vi "oa_Get DSA 9232 Oversample Rate and Filter Delay.vi"(11 "Requested Sample Rate":dbl) -> (0 "Decimation Rate":u16, 1 "Input Delay":dbl, 2 "Internal Master Timebase":dbl=13107200.0, 3 "Actual Sample Rate":dbl)   [LabVIEW 2017, in "SoundVib_TachProcess.lvlib"]
uses:
  <vilib>/addons/Sound and Vibration/Order Analysis/Tach Process/SoundVib_TachProcess.lvlib
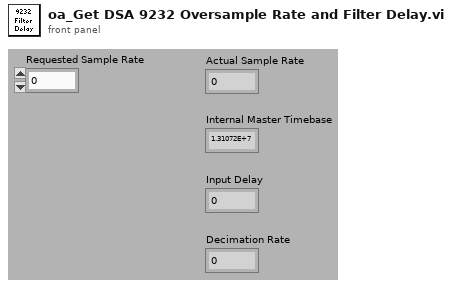
[diagram p1: front panel]
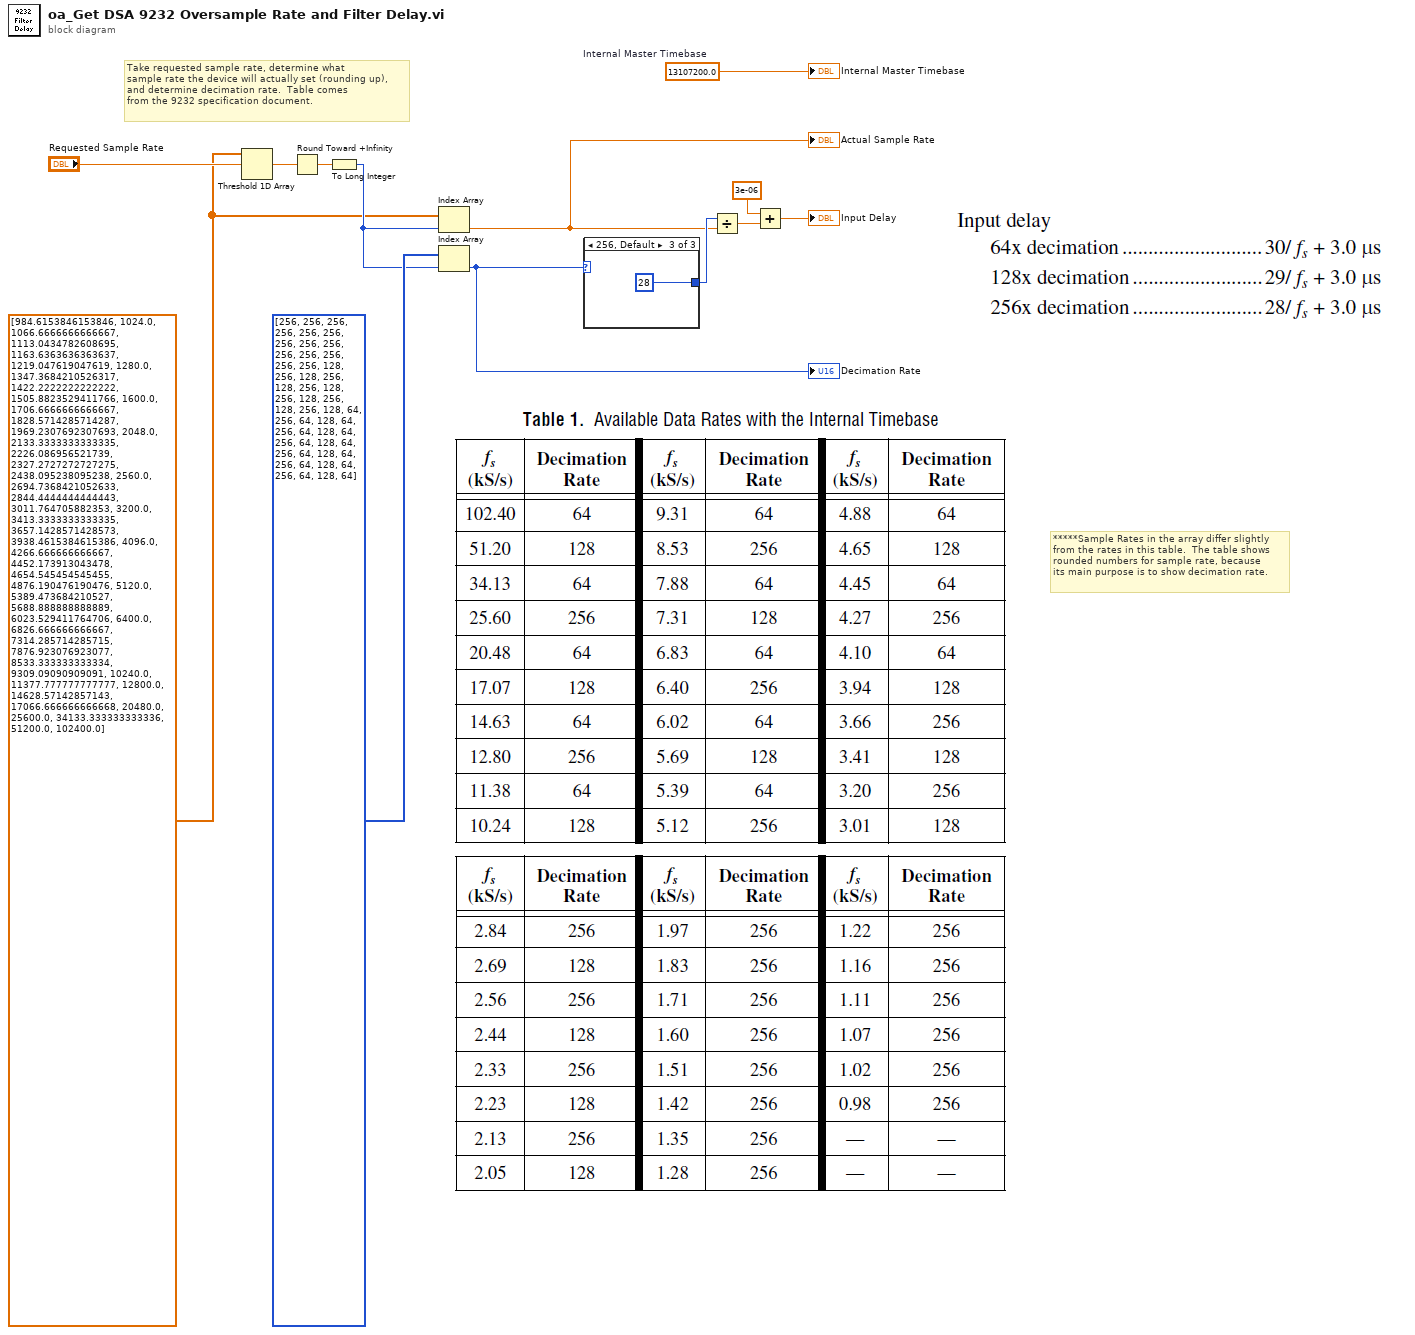
[diagram p0: block diagram]
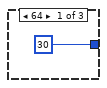
[diagram p2: hidden frame]
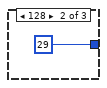
[diagram p3: hidden frame]
diagram:
  w1 = dbl[] [984.6153846153846, 1024.0, 1066.6666666666667, 1113.0434782608695, 1163.6363636363637, 1219.047619047619, 1280.0, 1347.3684210526317, 1422.2222222222222, 1505.8823529411766, 1600.0, 1706.6666666666667, 1828.5714285714287, 1969.2307692307693, 2048.0, 2133.3333333333335, 2226.086956521739, 2327.2727272727275, 2438.095238095238, 2560.0, 2694.7368421052633, 2844.4444444444443, 3011.764705882353, 3200.0, 3413.3333333333335, 3657.1428571428573, 3938.4615384615386, 4096.0, 4266.666666666667, 4452.173913043478, 4654.545454545455, 4876.190476190476, 5120.0, 5389.473684210527, 5688.888888888889, 6023.529411764706, 6400.0, 6826.666666666667, 7314.285714285715, 7876.923076923077, 8533.333333333334, 9309.09090909091, 10240.0, 11377.777777777777, 12800.0, 14628.57142857143, 17066.666666666668, 20480.0, 25600.0, 34133.333333333336, 51200.0, 102400.0] ("Possible Sample Rates")
  w2 = 13107200.0  # Internal Master Timebase
  # "*****Sample Rates in the array differ slightly\nfrom the rates in this table.  The table shows \nrounded numbers for sample rate, because\nits main purpose is to show decimation rate."
  # "Take requested sample rate, determine what\nsample rate the device will actually set (rounding up),\nand determine decimation rate.  Table comes\nfrom the 9232 specification document."
  n1 = Threshold 1D Array(2:"Requested Sample Rate", 3:w1) -> (0:w12:dbl)  [unwired: 1 in]
  n2 = Round Toward +Infinity(x=w12) -> (ceil(x): smallest int >= x=w10:dbl)
  n3 = To Long Integer(number=w10) -> (32bit integer=w9:i32)
  n4 = Index Array(array=w1, index=w9) -> (element=w6:dbl)
  "Actual Sample Rate" <- w6
  n5 = Index Array(array=u16[] [256, 256, 256, 256, 256, 256, 256, 256, 256, 256, 256, 256, 256, 256, 128, 256, 128, 256, 128, 256, 128, 256, 128, 256, 128, 256, 128, 64, 256, 64, 128, 64, 256, 64, 128, 64, 256, 64, 128, 64, 256, 64, 128, 64, 256, 64, 128, 64, 256, 64, 128, 64] ("reversed array"), index=w9) -> (element=w8:u16)
  "Decimation Rate" <- w8
  n6 = case shown="256, Default" w8 {
    tunnel: [30 29 28] -> w7
    frame 64 {
    }
    frame 128 {
    }
    frame 256, Default {
    }
  }
  n7 = Divide(x=w7, y=w6) -> (x/y=w5:dbl)
  n8 = Add(x=3e-06, y=w5) -> (x+y=→"Input Delay":dbl)
  "Internal Master Timebase" <- w2
